vi "Add Software Feed.vi"(6 "Trusted (F)":bool, 7 "Enabled (T)":bool=TRUE, 8 "error in (no error)":errorcluster, 9 "URI":string, 10 "Feed Name":string, 11 "Session in":refnum<k21>) -> (0 "error out":errorcluster, 3 "Session out":refnum<k21>)   [LabVIEW 2020, in "nisyscfg.lvlib"]
doc: "Adds a software feed to the system. This requires Secure Shell Server (sshd) to be enabled on the target."
uses:
  <vilib>/nisyscfg/nisyscfg.lvlib
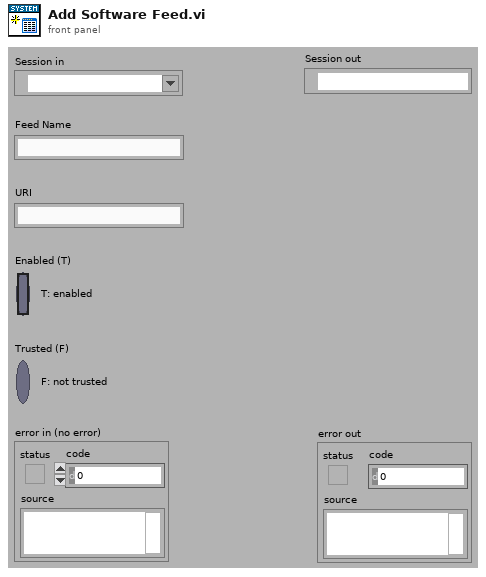
[diagram p1: front panel]
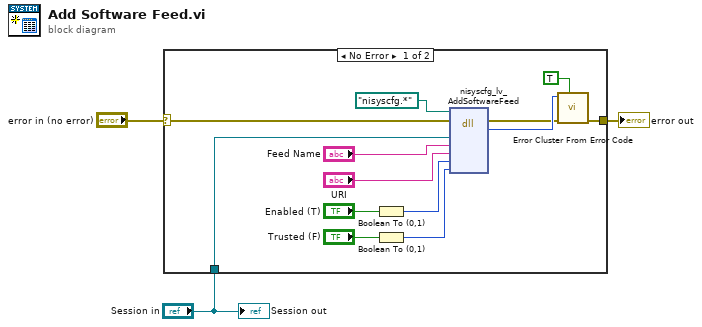
[diagram p0: block diagram]
diagram:
  n1 = case shown="No Error" "error in (no error)" {
    selector: "error in (no error)" -> [w11 w17]
    tunnel: [w12 w17] -> w3
    tunnel: "Session in" -> [w4 _]
    frame No Error {
      n2 = Boolean To (0,1)(Boolean="Enabled (T)") -> (0, 1=w8:i16)
      n3 = Boolean To (0,1)(Boolean="Trusted (F)") -> (0, 1=w7:i16)
      n4 = dll-call lib="nisyscfg.*" fn="nisyscfg_lv_AddSoftwareFeed" label="AddSoftwareFeed"(path in=path "nisyscfg.*", error in=w11, "sessionHandle"=w4, "feedName"="Feed Name", "uri"="URI", "enabled"=w8, "trusted"=w7) -> (error out=w15:errorcluster, "return type"=w16:i32)  [unwired: 6 in, 1 out]
      n5 = call <vilib>:"Error Cluster From Error Code.vi"("show call chain? (False)"=TRUE, "error in (no error)"=w15, "error code (0)"=w16) -> ("error out"=w12:errorcluster)  [unwired: 6 out]
    }
    frame Error {
    }
  }
  "error out" <- w3
  "Session out" <- "Session in"
